vi "Ex3_TempConversion.vi"() -> ()   [LabVIEW 2024]
panel:
  out "Kelvin":dbl(slide) scale=0.0..500.0
  out "Farenheit":dbl(slide) scale=0.0..200.0
  in  "Celsius":dbl(slide) scale=0.0..50.0
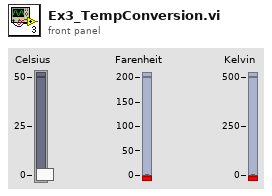
[diagram p1: front panel]
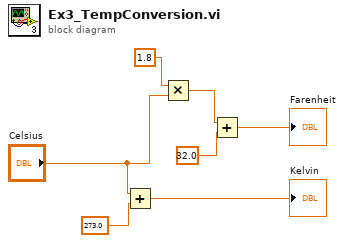
[diagram p0: block diagram]
diagram:
  n1 = Add(x="Celsius", y=273.0) -> (x+y=→"Kelvin":dbl)
  n2 = Multiply(x=1.8, y="Celsius") -> (x*y=w3:dbl)
  n3 = Add(x=w3, y=32.0) -> (x+y=→"Farenheit":dbl)
